vi "ExManualCalibWaveNumbers.vi"() -> ()   [LabVIEW 2010]
panel:
  in  "Stop":bool
  in  "Finished picking peaks":bool
  out "XY Graph":cluster{dbl[], "Array i32":i32[]}(graph)
  in  "Wavelength 3":dbl=576.96 format="%.2f"
  in  "Pixel 3":dbl=537.0 format="%.2f"
  in  "Wavelength 2":dbl=546.074 format="%.2f"
  in  "Pixel 2":dbl=485.0 format="%.2f"
  in  "Wavelength 1":dbl=435.833 format="%.2f"
  in  "Pixel 1":dbl=301.0 format="%.2f"
  out "error out":errorcluster
  in  "error in (no error)":errorcluster
  in  "FileType":u32=67174400
  in  "Full File Name":path=path "C:/Program Files/SIToolKit/LabVIEW/Data Files/HID-LAMP.TIF"
  # "ExManualCalibWaveNumbers.vi : this example shows\nhow to do a manual calibration with the result in wavenumbers. \nFirst select a file with data in it with know peaks (i.e. mercury \nlamp). then start VI. Enter pixel of peak with what wavelength \npeak should be. This example does three peaks, but more can \nbe used if available. Once all pixels and wavelengths have been\nentered then hit the finished button. The displahy will\nnow show a calibrated data with wavelength on the \nx axis. The cursor can be moved around to verify\nthe calibration. Hit stop button when done with calibration.\nUser may want to save calibration points in ascii file so that \nthese values can be used when collecting live data."
  # "File Types:\nSPE = 67371008\nTIF   = 67174400\nPMI  = 67436544"
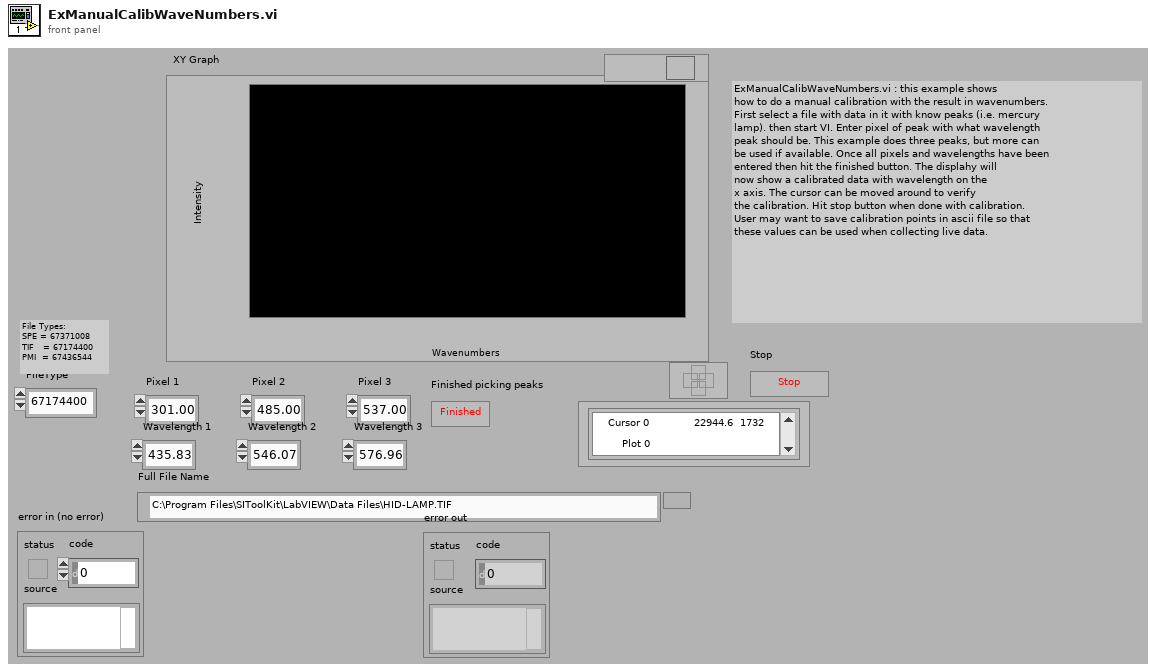
[diagram p1: front panel]
types:
  T1 = cluster{"total pairs":i32, "Order of\nPolynominal":i32, "Units in\n4-nm":i32, "Output units\n4-nm, 5 wavenumbers":i32, "Laser line wavelength in nm":dbl}
  T2 = cluster{"Calibrated Array":dbl[], "Array i32":i32[]}
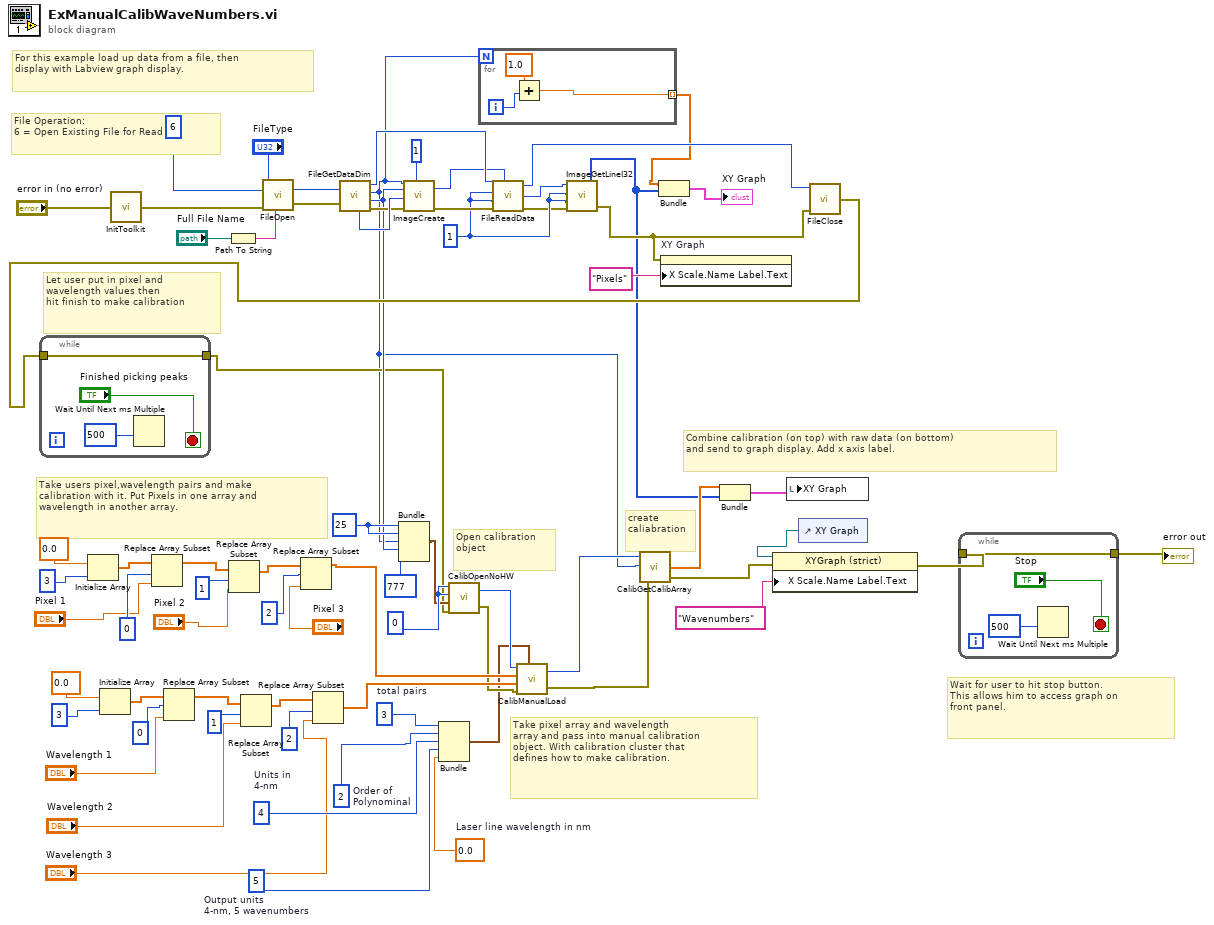
[diagram p0: block diagram]
diagram:
  w22 = 0.0  # Laser line wavelength in nm
  w23 = 5  # Output units 4-nm, 5 wavenumbers
  w24 = 4  # Units in 4-nm
  w25 = 2  # Order of Polynominal
  w26 = 3  # total pairs
  w27 = 0
  w29 = 25
  w58 = 1
  # "Wait for user to hit stop button.\nThis allows him to access graph on\nfront panel."
  # "Combine calibration (on top) with raw data (on bottom) \nand send to graph display. Add x axis label."
  # "create \ncaliabration"
  # "Open calibration\nobject"
  # "Take pixel array and wavelength \narray and pass into manual calibration \nobject. With calibration cluster that \ndefines how to make calibration."
  # "Take users pixel,wavelength pairs and make \ncalibration with it. Put Pixels in one array and\nwavelength in another array."
  # "Let user put in pixel and \nwavelength values then \nhit finish to make calibration"
  # "For this example load up data from a file, then\ndisplay with Labview graph display."
  # "File Operation:\n6 = Open Existing File for Read"
  n1 = Initialize Array(0.0, 3) -> (w46:dbl[])
  n2 = Initialize Array(0.0, 3) -> (w39:dbl[])
  n3 = call <userlib>:"InitToolkit.vi"("error in"="error in (no error)") -> ("error out"=w70:errorcluster)
  n4 = Replace Array Subset(array=w46, new element="Pixel 1", index=0) -> (w45:dbl[])
  n5 = Replace Array Subset(array=w39, new element="Wavelength 1", index=0) -> (w38:dbl[])
  n6 = Path To String(path="Full File Name") -> (string=w64:string)
  n7 = Replace Array Subset(array=w45, new element="Pixel 2", index=1) -> (w44:dbl[])
  n8 = Replace Array Subset(array=w38, new element="Wavelength 2", index=1) -> (w37:dbl[])
  n9 = call <userlib>:"FileOpen.vi"("error in"=w70, "File Operations"=u32 6 ("File Operation"), "FileName"=w64, "File Type"="FileType") -> ("error out"=w68:errorcluster, "File Handle"=w67:u32)
  n10 = Replace Array Subset(array=w44, new element="Pixel 3", index=2) -> (w32:dbl[])
  n11 = Replace Array Subset(array=w37, new element="Wavelength 3", index=2) -> (w33:dbl[])
  n12 = call <userlib>:"FileGetDataDim.vi"("File Handle"=w67, "error in"=w68) -> ("Data Type"=w56:u32, "File Handle"=w61:u32, "X dim"=w9:u32, "Y dim"=w14:u32, "error out"=w55:errorcluster)  [unwired: 1 out]
  n13 = Bundle(w29, w29, "X dim"=w9, "Y dim"=w14, 777) -> (w13:cluster{i32, i32, "X dim":u32, "Y dim":u32, i32})  [unwired: 1 in]
  n14 = call <userlib>:"ImageCreate.vi"("X dimension"=w9, "Y dimension"=w14, "Data Type"=w56, "error in"=w55, "Number Of Frames"=1) -> ("Image Handle"=w60:u32, "error out"=w63:errorcluster)
  n15 = Bundle("total pairs"=w26, "Order of\nPolynominal"=w25, "Units in\n4-nm"=w24, "Output units\n4-nm, 5 wavenumbers"=w23, "Laser line wavelength in nm"=w22) -> (w21:T1)  [unwired: 1 in]
  n16 = for {
    N: w9 -> [_]
    tunnel: [w73] -> w54 mode=indexing
    i -> [w74]
    n17 = Add(x=1.0, y=w74) -> (x+y=w73:dbl)
  }
  n18 = call <userlib>:"FileReadData.vi"("File Handle"=w61, "Start Frame"=w58, "End Frame"=w58, "error in"=w63, "Image Handle"=w60) -> ("File Handle"=w59:u32, "Image Handle"=w62:u32, "error out"=w57:errorcluster)
  n19 = call <userlib>:"ImageGetLineI32.vi"("error in"=w57, "Z Position"=w58, "Y Position"=w58, "Data Handle"=w62) -> ("error out"=w51:errorcluster, "Array i32"=w1:i32[])  [unwired: 1 out]
  n20 = Bundle(w54, "Array i32"=w1) -> (→"XY Graph":cluster{dbl[], "Array i32":i32[]})  [unwired: 1 in]
  n21 = property on="XY Graph" class="XYGraph (strict)"(error in=w51, "X Scale.Name Label.Text"="Pixels") -> ()  [unwired: 1 in, 2 out]
  n22 = control-ref of="XY Graph"() -> (w4:refnum<vi>)
  n23 = call <userlib>:"FileClose.vi"("error in"=w51, "File Handle"=w59) -> ("error out"=w50:errorcluster)
  n24 = while {
    tunnel: w50 -> [w77]
    tunnel: [w77] -> w12
    stop <- "Finished picking peaks" stop-if-true
    n25 = Wait Until Next ms Multiple(millisecond multiple=500) -> ()  [unwired: 1 out]
  }
  n26 = call <userlib>:"CalibOpenNoHW.vi"("error in"=w12, "Data Info"=w13, "Calibration Type"=w27, "Calibration Device ID"=w27) -> ("error out"=w30:errorcluster, "Calibration Handle"=w31:u32)
  n27 = call <userlib>:"CalibManualLoad.vi"("Calibration Handle"=w31, "Pixel Array"=w32, "Wavelength Array"=w33, "error in (no error)"=w30, "Calibration Values"=w21) -> ("Calibration Handle"=w10:u32, "error out"=w11:errorcluster)
  n28 = call <userlib>:"CalibGetCalibArray.vi"("error in"=w11, "Array Size"=w9, "Calibration Handle"=w10) -> ("error out"=w6:errorcluster, "Calibrated Array"=w2:dbl[])  [unwired: 1 out]
  n29 = Bundle("Calibrated Array"=w2, "Array i32"=w1) -> (w8:T2)  [unwired: 1 in]
  n30 = property on="Property Node" class="XYGraph (strict)"(reference=w4, error in=w6, "X Scale.Name Label.Text"="Wavenumbers") -> (error out=w5:errorcluster)  [unwired: 1 out]
  n31 = local write "XY Graph"(w8) -> ()
  n32 = while {
    tunnel: w5 -> [w80]
    tunnel: [w80] -> w7
    stop <- "Stop" stop-if-true
    n33 = Wait Until Next ms Multiple(millisecond multiple=500) -> ()  [unwired: 1 out]
  }
  "error out" <- w7
